vi "Actor Core.vi"(8 "error in":errorcluster, 11 "DAQmx Recorder in":refnum<class "DAQmx Recorder.lvclass">) -> (0 "error out":errorcluster, 3 "Actor out":refnum<class "Actor.lvclass">)   [LabVIEW 2015, in "DAQmx Recorder.lvclass"]
doc: "(<B>Filename</B>: Actor Framework.lvlib:Actor.lvclass:Actor Core.vi)\n\nReceives messages to the actor, reacts to them, and initiates any error handling that may shut the actor down.\n\nDescendant classes may override this VI to append parallel tasks for the actor to complete while it handles messages. Overrides use the Call Parent Method node."
uses:
  DAQmx Recorder.lvclass
  <vilib>/ActorFramework/Actor/Actor.lvclass
  NHMFL_Core/Libraries/NI-DAQ/DAQmx Digitizer/DAQmx Digitizer Configuration.ctl
  Measure_core/Pulse Recorders/Pulse Recorder/Pulse Recorder.lvclass
panel:
  in  "Configuration":T1={"Pre-trigger duration"=0.01, "Post-trigger duration"=0.1, "Rate"=1000000.0, "Range"=10.0, "Physical Channels"="", "input configuration"=-1, "Channel names"=["Bdot", "Idot"]} {"input configuration" items=["Default"=-1, "RSE"=10083, "NRSE"=10078, "Differential"=10106, "Pseudodifferential"=12529]; "Rate" format="%#_6pHz"; "Post-trigger duration" format="%#_6ps"; "Pre-trigger duration" format="%#_6ps"; "Range" format="%#_6pV"}
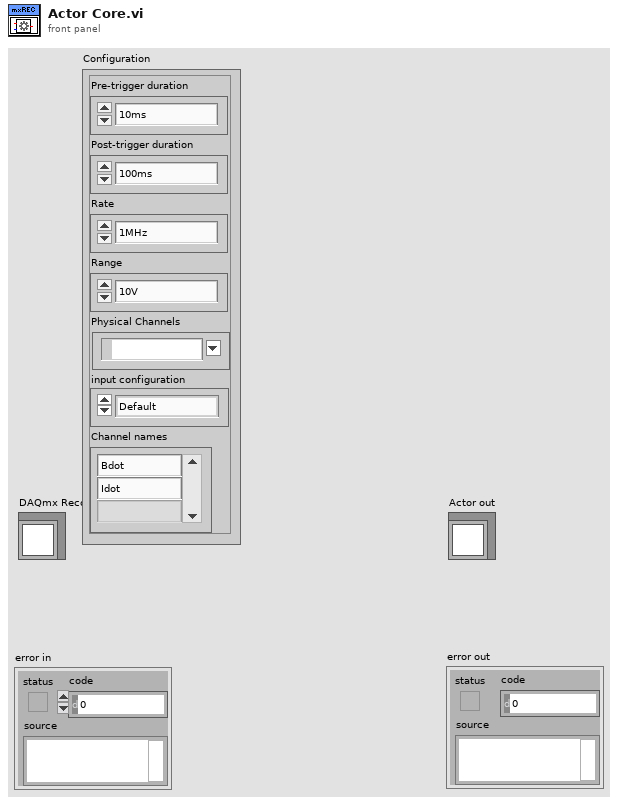
[diagram p1: front panel]
types:
  T1 = typedef "DAQmx Digitizer Configuration.ctl" = cluster{"Pre-trigger duration":dbl, "Post-trigger duration":dbl, "Rate":dbl, "Range":dbl, "Physical Channels":tag, "input configuration":i32, "Channel names":string[]}
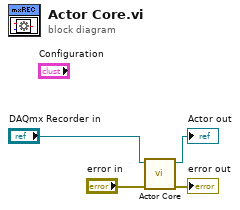
[diagram p0: block diagram]
diagram:
  n1 = call-parent "Actor Core.vi"("error in"="error in", "Measure Object in"="DAQmx Recorder in") -> ("error out"=→"error out":errorcluster, "Actor out"=→"Actor out":refnum<class "Actor.lvclass">)  [unwired: 8 in]
